vi "Setup New Round.vi"(8 "Team Index":i32, 9 "Round":i32, 10 "Board Size":i32, 11 "Global Data":T1) -> (3 "Global Data Out":T1, 5 "Data.Order ID Out":i32)   [LabVIEW 2017, in "AntFarm_MB.lvclass"]
uses:
  AntFarm_MB.lvclass
  TypeDefs/Cluster_Ant Farm Global Data.ctl
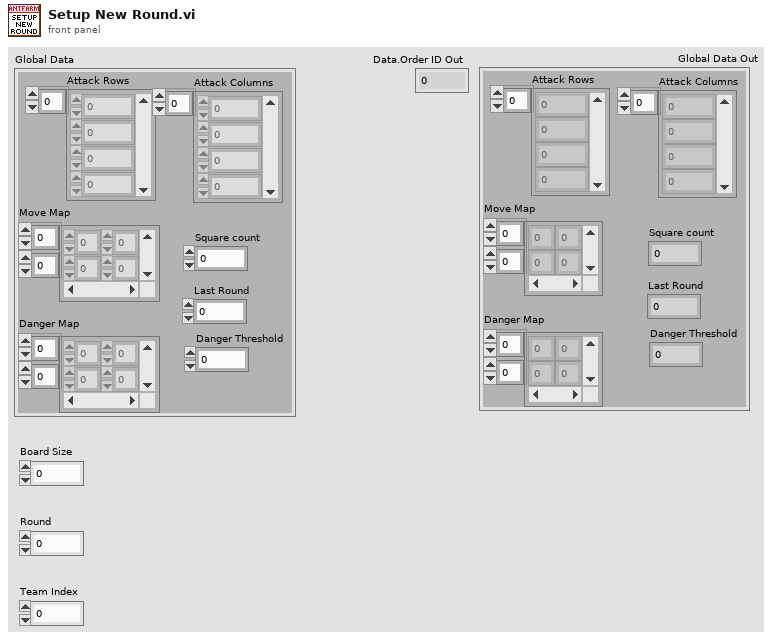
[diagram p1: front panel]
types:
  T1 = typedef "Cluster_Ant Farm Global Data.ctl" = cluster{"Move Map":i32[][], "Danger Map":i32[][], "Attack Rows":i32[], "Attack Columns":i32[], "Square count":i32, "Last Round":i32, "Danger Threshold":i32}
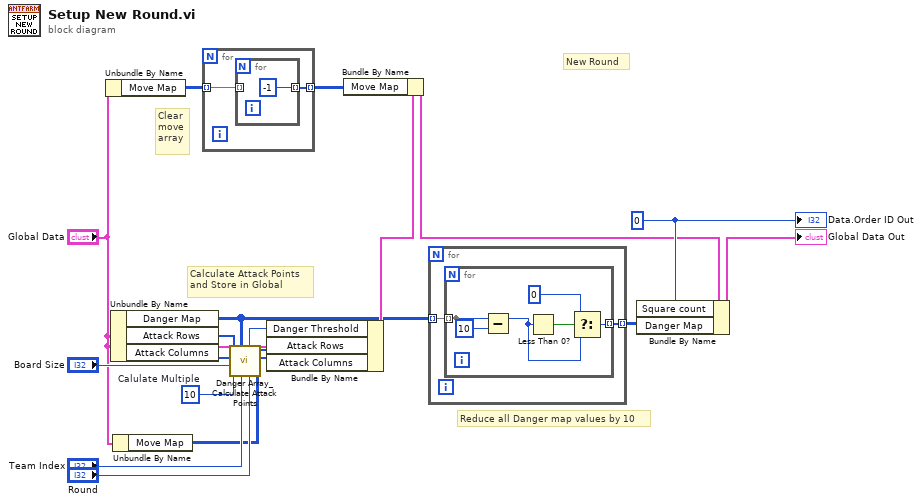
[diagram p0: block diagram]
diagram:
  w4 = 10  # Calulate Multiple
  w15 = 0 ("Data.Order ID")
  # "Calculate Attack Points\nand Store in Global"
  # "Reduce all Danger map values by 10"
  # "Clear \nmove\narray"
  # "New Round"
  n1 = Unbundle By Name("Global Data") -> ("Move Map"=w6:i32[][])
  n2 = Unbundle By Name("Global Data") -> ("Danger Map"=w5:i32[][], "Attack Rows"=w18:i32[], "Attack Columns"=w19:i32[])
  n3 = Unbundle By Name("Global Data") -> ("Move Map"=w1:i32[][])
  n4 = for {
    tunnel: w6 -> [w21] mode=indexing
    tunnel: [w20] -> w7 mode=indexing
    n5 = for {
      tunnel: w21 -> [_] mode=indexing
      tunnel: [-1] -> w20 mode=indexing
    }
  }
  n6 = call "Danger Array_Calculate Attack Points.vi"("Move Map"=w1, "Round"="Round", "Team Index"="Team Index", "Danger Map"=w5, "Calulate Multiple"=w4, "Board Size"="Board Size", "Danger Column"=w19, "Danger Row"=w18) -> ("Danger Column Out"=w11:i32[], "Danger Row Out"=w10:i32[], "Danger Threshold"=w3:i32)  [unwired: 1 in]
  n7 = Bundle By Name(cluster="Global Data", "Danger Threshold"=w3, "Attack Rows"=w10, "Attack Columns"=w11) -> (w9:T1)
  n8 = Bundle By Name(cluster=w9, "Move Map"=w7) -> (w12:T1)
  n9 = for {
    tunnel: w5 -> [w23] mode=indexing
    tunnel: [w24] -> w14 mode=indexing
    tunnel: [w23] -> _ mode=indexing
    n10 = for {
      tunnel: w23 -> [w27] mode=indexing
      tunnel: [w28] -> w24 mode=indexing
      n11 = Subtract(x=w27, y=10) -> (x-y=w26:i32)
      n12 = Less Than 0?(x=w26) -> (x < 0?=w30:bool)
      n13 = Select(t=0 ("Round"), s=w30, f=w26) -> (s? t:f=w28:i32)
    }
  }
  n14 = Bundle By Name(cluster=w12, "Square count"=w15, "Danger Map"=w14) -> (→"Global Data Out":T1)
  "Data.Order ID Out" <- w15
